vi "ErwKonf_PID_SysLog.vi"(11 "NewVal":T1 {"Heizung\nFB-Druckregler"."max. OUT" format="%#_5g"; "Heizung\nFB-Druckregler"."Regelzonengr." format="%#_5g"; "Heizung\nFB-Druckregler"."D-Anteil" format="%#_5g"; "Heizung\nFB-Druckregler"."I-Anteil" format="%#_5g"; "Heizung\nFB-Druckregler"."P-Anteil" format="%.1f"; "Heizleitung\nExtern"."max. OUT" format="%#_5g"; "Heizleitung\nExtern"."Regelzonengr." format="%#_5g"; "Heizleitung\nExtern"."D-Anteil" format="%#_5g"; "Heizleitung\nExtern"."I-Anteil" format="%#_5g"; "Heizleitung\nExtern"."P-Anteil" format="%.1f"; "Heizung\nHeizleitungen"."max. OUT" format="%#_5g"; "Heizung\nHeizleitungen"."Regelzonengr." format="%#_5g"; "Heizung\nHeizleitungen"."D-Anteil" format="%#_5g"; "Heizung\nHeizleitungen"."I-Anteil" format="%#_5g"; "Heizung\nHeizleitungen"."P-Anteil" format="%.1f"; "Heizung\nPumpe"."max. OUT" format="%#_5g"; "Heizung\nPumpe"."Regelzonengr." format="%#_5g"; "Heizung\nPumpe"."D-Anteil" format="%#_5g"; "Heizung\nPumpe"."I-Anteil" format="%#_5g"; "Heizung\nPumpe"."P-Anteil" format="%.1f"; "Heizung\nFilterblock"."max. OUT" format="%#_5g"; "Heizung\nFilterblock"."Regelzonengr." format="%#_5g"; "Heizung\nFilterblock"."D-Anteil" format="%#_5g"; "Heizung\nFilterblock"."I-Anteil" format="%#_5g"; "Heizung\nFilterblock"."P-Anteil" format="%.1f"}) -> (3 "NewVal out":T1 {"Heizung\nFB-Druckregler"."max. OUT" format="%#_5g"; "Heizung\nFB-Druckregler"."Regelzonengr." format="%#_5g"; "Heizung\nFB-Druckregler"."D-Anteil" format="%#_5g"; "Heizung\nFB-Druckregler"."I-Anteil" format="%#_5g"; "Heizung\nFB-Druckregler"."P-Anteil" format="%.1f"; "Heizleitung\nExtern"."max. OUT" format="%#_5g"; "Heizleitung\nExtern"."Regelzonengr." format="%#_5g"; "Heizleitung\nExtern"."D-Anteil" format="%#_5g"; "Heizleitung\nExtern"."I-Anteil" format="%#_5g"; "Heizleitung\nExtern"."P-Anteil" format="%.1f"; "Heizung\nHeizleitungen"."max. OUT" format="%#_5g"; "Heizung\nHeizleitungen"."Regelzonengr." format="%#_5g"; "Heizung\nHeizleitungen"."D-Anteil" format="%#_5g"; "Heizung\nHeizleitungen"."I-Anteil" format="%#_5g"; "Heizung\nHeizleitungen"."P-Anteil" format="%.1f"; "Heizung\nPumpe"."max. OUT" format="%#_5g"; "Heizung\nPumpe"."Regelzonengr." format="%#_5g"; "Heizung\nPumpe"."D-Anteil" format="%#_5g"; "Heizung\nPumpe"."I-Anteil" format="%#_5g"; "Heizung\nPumpe"."P-Anteil" format="%.1f"; "Heizung\nFilterblock"."max. OUT" format="%#_5g"; "Heizung\nFilterblock"."Regelzonengr." format="%#_5g"; "Heizung\nFilterblock"."D-Anteil" format="%#_5g"; "Heizung\nFilterblock"."I-Anteil" format="%#_5g"; "Heizung\nFilterblock"."P-Anteil" format="%.1f"})   [LabVIEW 2020, in "Erweiterte Konfig.lvlib"]
uses:
  Erweiterte Konfig.lvlib
  PID-Parameter Anzeige.ctl
  PID-Parameter.ctl
  Visualisierungs Elemente/Zahlen-Eingabefeld.ctl
  FGV PID Aktionen.ctl
panel:
  # "sec"
  # "sec"
  # "°C"
  # "%"
  # "sec"
  # "sec"
  # "°C"
  # "%"
  # "sec"
  # "sec"
  # "°C"
  # "%"
  # "sec"
  # "sec"
  # "°C"
  # "%"
  # "sec"
  # "sec"
  # "°C"
  # "%"
  # "sec"
  # "sec"
  # "°C"
  # "%"
  # "sec"
  # "sec"
  # "°C"
  # "%"
  # "sec"
  # "sec"
  # "°C"
  # "%"
  # "sec"
  # "sec"
  # "°C"
  # "%"
  # "sec"
  # "sec"
  # "°C"
  # "%"
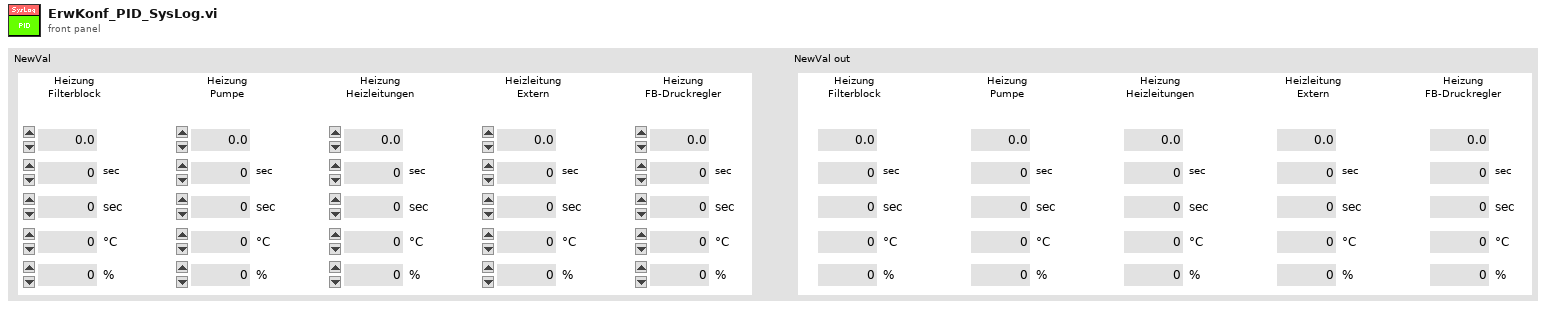
[diagram p1: front panel]
types:
  T1 = typedef "Erweiterte Konfig.lvlib/PID-Parameter Anzeige.ctl" = cluster{"Heizung\nFilterblock":T2, "Heizung\nPumpe":T2, "Heizung\nHeizleitungen":T2, "Heizleitung\nExtern":T2, "Heizung\nFB-Druckregler":T2}
  T2 = typedef "Erweiterte Konfig.lvlib/PID-Parameter.ctl" = cluster{"P-Anteil":T3, "I-Anteil":T3, "D-Anteil":T3, "Regelzonengr.":T3, "max. OUT":T3}
  T3 = typedef "Zahlen-Eingabefeld.ctl" = sgl
  T4 = typedef "Erweiterte Konfig.lvlib/FGV PID Aktionen.ctl" = enum16{"Lesen", "Schreiben PID", "Schreiben Sonstige", "Dichtheitstest", "Aktionen Dicht.", "Parameter Sensor"}
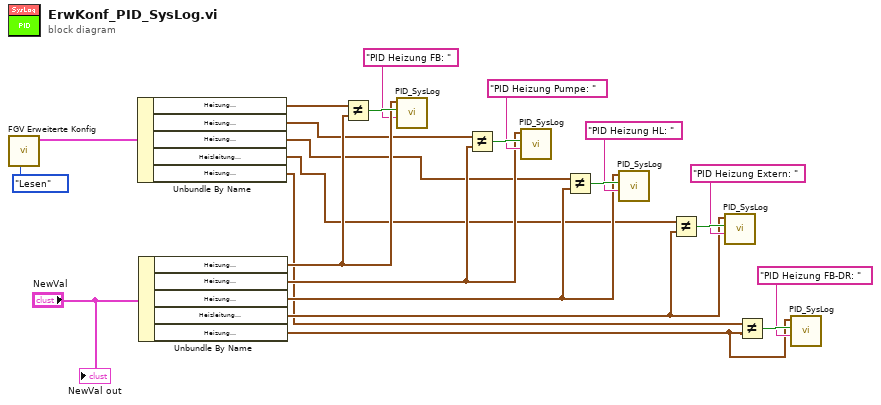
[diagram p0: block diagram]
diagram:
  n1 = call "FGV Erweiterte Konfig.vi"("Aktion"=FGV_PID_Aktionen."Lesen") -> ("PID-Parameter Anzeige"=w22:T1)  [unwired: 5 in, 5 out]
  n2 = Unbundle By Name(w22) -> ("Heizung\nFilterblock"=w20:T2, "Heizung\nPumpe"=w8:T2, "Heizung\nHeizleitungen"=w4:T2, "Heizleitung\nExtern"=w3:T2, "Heizung\nFB-Druckregler"=w2:T2)
  n3 = Unbundle By Name("NewVal") -> ("Heizung\nFilterblock"=w18:T2, "Heizung\nPumpe"=w7:T2, "Heizung\nHeizleitungen"=w6:T2, "Heizleitung\nExtern"=w5:T2, "Heizung\nFB-Druckregler"=w1:T2)
  n4 = Not Equal?(x=w20, y=w18) -> (x != y?=w19:bool)
  n5 = call "PID_SysLog.vi"("Fehlermeldung"="PID Heizung FB: ", "Boolesch"=w19, "Heizung\nFilterblock"=w18) -> ()  [unwired: 9 in]
  n6 = Not Equal?(x=w8, y=w7) -> (x != y?=w16:bool)
  n7 = call "PID_SysLog.vi"("Fehlermeldung"="PID Heizung Pumpe: ", "Boolesch"=w16, "Heizung\nFilterblock"=w7) -> ()  [unwired: 9 in]
  n8 = Not Equal?(x=w4, y=w6) -> (x != y?=w14:bool)
  n9 = call "PID_SysLog.vi"("Fehlermeldung"="PID Heizung HL: ", "Boolesch"=w14, "Heizung\nFilterblock"=w6) -> ()  [unwired: 9 in]
  n10 = Not Equal?(x=w3, y=w5) -> (x != y?=w12:bool)
  n11 = call "PID_SysLog.vi"("Fehlermeldung"="PID Heizung Extern: ", "Boolesch"=w12, "Heizung\nFilterblock"=w5) -> ()  [unwired: 9 in]
  n12 = Not Equal?(x=w2, y=w1) -> (x != y?=w10:bool)
  n13 = call "PID_SysLog.vi"("Fehlermeldung"="PID Heizung FB-DR: ", "Boolesch"=w10, "Heizung\nFilterblock"=w1) -> ()  [unwired: 9 in]
  "NewVal out" <- "NewVal"
